vi "Avg Tovey Force Data.vi"(0 "Model in":refnum<class "Model.lvclass">, 5 "After This Time":dbl, 11 "error in (no error)":errorcluster) -> (4 "Model out":refnum<class "Model.lvclass">, 6 "Fz":dbl, 8 "Fy":dbl, 10 "Fx":dbl, 15 "error out":errorcluster)   [LabVIEW 2016, in "Model.lvclass"]
uses:
  Model.lvclass
  Model.lvclass/Model.ctl
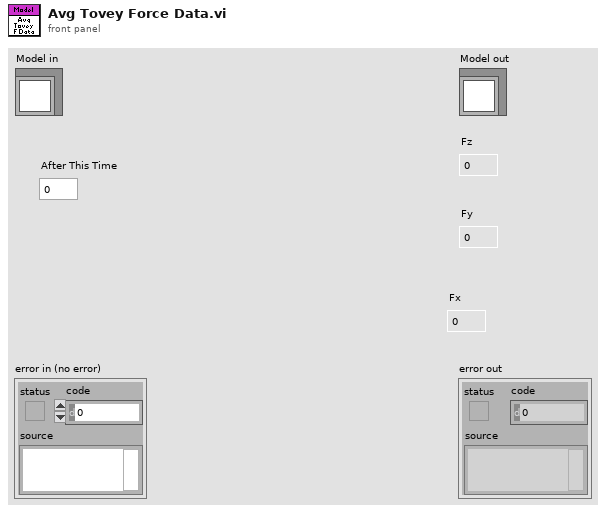
[diagram p1: front panel]
types:
  T1 = typedef "FAMT Typedefs.lvlib/ToveyEngData.ctl" = cluster{"Timestamp":dbl, "Fx":dbl, "Fy":dbl, "Fz":dbl, "Mx":dbl, "My":dbl, "Mz":dbl}
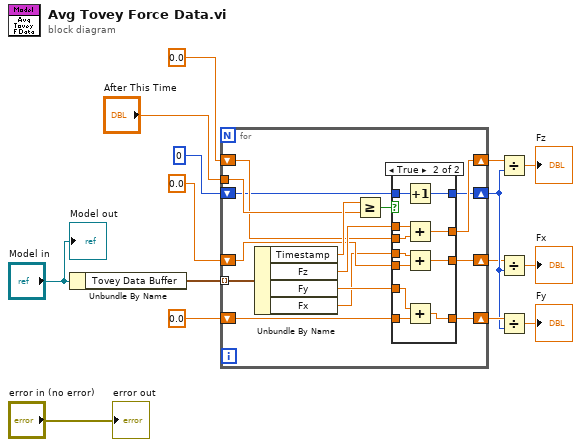
[diagram p0: block diagram]
diagram:
  n1 = Unbundle By Name("Model in") -> ("Tovey Data Buffer"=w15:T1[])
  n2 = for {
    tunnel: w15 -> [w30] mode=indexing
    tunnel: "After This Time" -> [w28]
    shift-right: [w25] -> w10
    shift-left: 0.0 -> [w24]
    shift-right: [w22] -> w2
    shift-left: 0 -> [w23]
    shift-right: [w20] -> w9
    shift-left: 0.0 -> [w19]
    shift-right: [w17] -> w1
    shift-left: 0.0 -> [w18]
    n3 = Unbundle By Name(w30) -> ("Timestamp"=w29:dbl, "Fz"=w26:dbl, "Fy"=w21:dbl, "Fx"=w16:dbl)
    n4 = Greater Or Equal?(x=w29, y=w28) -> (x >= y?=w27:bool)
    n5 = case shown="True" w27 {
      tunnel: w26 -> [_ w45]
      tunnel: [w33 w44] -> w25
      tunnel: w24 -> [w33 w43]
      tunnel: w23 -> [w34 w42]
      tunnel: [w34 w41] -> w22
      tunnel: w21 -> [_ w40]
      tunnel: [w32 w39] -> w20
      tunnel: w19 -> [w32 w38]
      tunnel: w18 -> [w31 w37]
      tunnel: [w31 w36] -> w17
      tunnel: w16 -> [_ w35]
      frame False {
      }
      frame True {
        n6 = Increment(x=w42) -> (x+1=w41:i32)
        n7 = Add(x=w45, y=w43) -> (x+y=w44:dbl)
        n8 = Add(x=w35, y=w37) -> (x+y=w36:dbl)
        n9 = Add(x=w40, y=w38) -> (x+y=w39:dbl)
      }
    }
  }
  n10 = Divide(x=w10, y=w2) -> (x/y=→"Fz":dbl)
  n11 = Divide(x=w1, y=w2) -> (x/y=→"Fx":dbl)
  n12 = Divide(x=w9, y=w2) -> (x/y=→"Fy":dbl)
  "error out" <- "error in (no error)"
  "Model out" <- "Model in"
